vi "Do.vi"(8 "error in (no error)":errorcluster, 10 "Actor in":refnum<class "Actor.lvclass">, 11 "Global Reset Msg":refnum<class "Global Reset Msg.lvclass">) -> (0 "error out":errorcluster, 2 "Actor out":refnum<class "Actor.lvclass">)   [LabVIEW 2023, in "GUI.lvlib" / "Diagnostic.lvlib" / "Global Reset Msg.lvclass"]
doc: "This VI delivers the message to the actor by calling the appropriate method(s) on the actor."
uses:
  Global Reset Msg.lvclass
  <vilib>/ActorFramework/Actor/Actor.lvclass
  Global Reset Msg.lvclass/Global Reset Msg.ctl
  Diagnostic/Diagnostic.lvclass
  d0cfc196-07c1-4e47-8cad-3cd91778ebab.vi
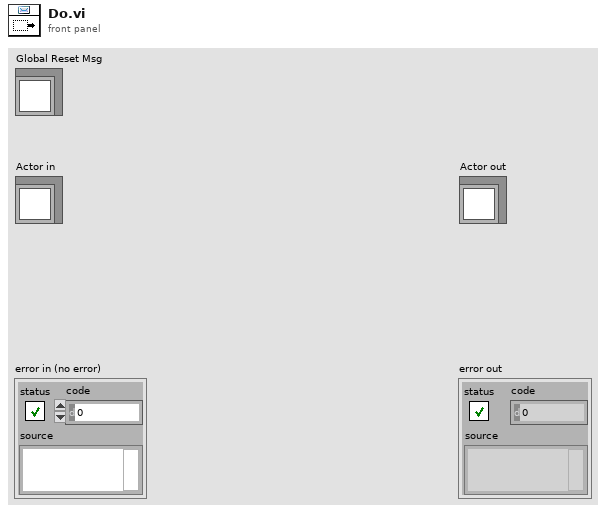
[diagram p1: front panel]
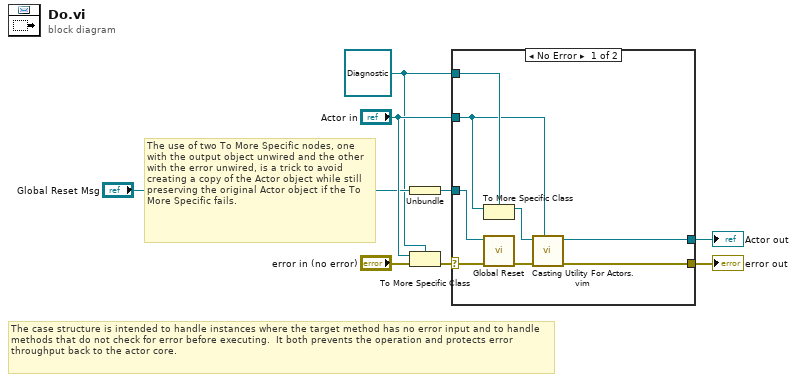
[diagram p0: block diagram]
diagram:
  w3 = refnum<class "Diagnostic.lvclass"> refnum ("Actor in")
  # "The use of two To More Specific nodes, one with the output object unwired and the other with the error unwired, is a trick to avoid creating a copy of the Actor object while still preserving the original Actor object if the To More Specific fails."
  # "The case structure is intended to handle instances where the target method has no error input and to handle methods that do not check for error before executing.  It both prevents the operation and protects error throughput back to the actor core."
  n1 = Unbundle("Global Reset Msg") -> (w1:refnum<vi>)
  n2 = To More Specific Class(target class=w3, reference="Actor in", error in="error in (no error)") -> (error out=w2:errorcluster)  [unwired: 1 out]
  n3 = case shown="No Error" w2 {
    selector: w2 -> [w16 w18]
    tunnel: [w11 w18] -> w8
    tunnel: [w12 w17] -> w7
    tunnel: "Actor in" -> [w13 w17]
    tunnel: w3 -> [w14 _]
    tunnel: w1 -> [w9 _]
    frame No Error {
      n4 = To More Specific Class(target class=w14, reference=w13) -> (specific class reference=w15:refnum<class "Diagnostic.lvclass">)  [unwired: 1 in, 1 out]
      n5 = call "Global Reset.vi"("error in"=w16, "Clobal Reset"=w9) -> ("error out"=w10:errorcluster)  [unwired: 9 in]
      n6 = call "Casting Utility For Actors.vim"("type"=w13, "error in (no error)"=w10, "Actor in"=w15) -> ("error out"=w11:errorcluster, "Actor out"=w12:refnum<class "Actor.lvclass">)  [unwired: 7 in]
    }
    frame Error {
      # "If type check fails, pass the original object out again."
    }
  }
  "error out" <- w8
  "Actor out" <- w7
